vi "De-Initialize.vi"(8 "error in (no error)":errorcluster, 11 "ZI Lockin in":refnum<class "ZI Lockin.lvclass">) -> (0 "error out":errorcluster, 3 "ZI Lockin out":refnum<class "ZI Lockin.lvclass">)   [LabVIEW 2017, in "ZI Lockin.lvclass"]
uses:
  ZI Lockin.lvclass
  ZI Lockin.lvclass/ZI Lockin.ctl
  Read ZI Handle.vi
  Write ZI Handle.vi
  <instrlib>/Zurich Instruments LabOne/Zurich Instruments LabOne.lvlib
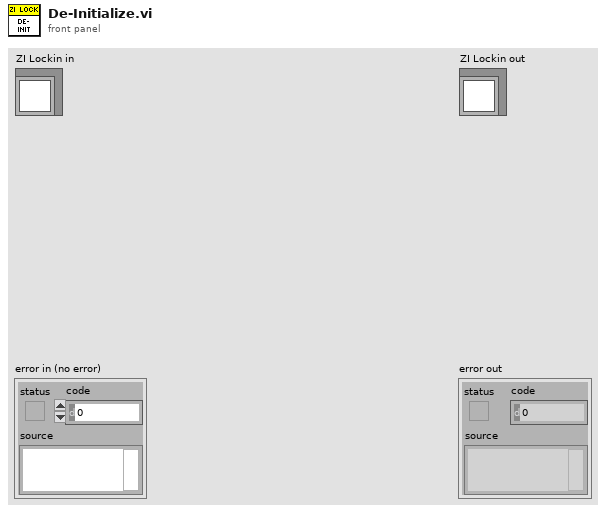
[diagram p1: front panel]
types:
  T1 = typedef "Zurich Instruments LabOne.lvlib/ziTypeHandle.ctl" = cluster{"handleValid":bool, "Conn":u64, "Path Prefix":string, "Handle":u64, "Connected":bool, "Clockbase(s)":dbl}
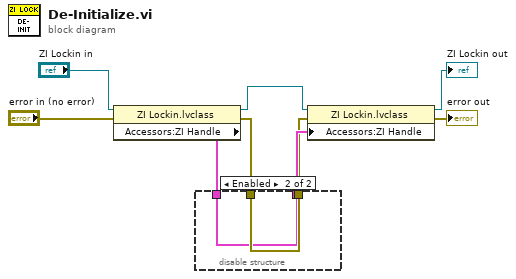
[diagram p0: block diagram]
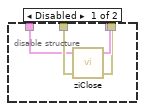
[diagram p2: hidden frame]
diagram:
  n1 = property class="ZI Lockin.lvclass"(reference="ZI Lockin in", error in="error in (no error)") -> (reference out=w9:refnum<class "ZI Lockin.lvclass">, error out=w7:errorcluster, "Accessors:ZI Handle"=w1:T1)
  n2 = disable-structure shown="Enabled" {
    disable-tunnel: [w13 w14] -> w8
    disable-tunnel: w7 -> [w12 w15]
    disable-tunnel: [w11 w15] -> w6
    disable-tunnel: w1 -> [w10 w14]
    frame Disabled {
      n3 = call <instrlib>:"ziClose.vi"("Error In"=w12, "Handle In"=w10) -> ("Error Out"=w11:errorcluster, "Handle Out"=w13:T1)  [unwired: 2 in]
    }
    frame Enabled {
    }
  }
  n4 = property class="ZI Lockin.lvclass"(reference=w9, error in=w6, "Accessors:ZI Handle"=w8) -> (reference out=→"ZI Lockin out":refnum<class "ZI Lockin.lvclass">, error out=→"error out":errorcluster)
